vi "ADI_IMU_ADIS16448_ScaleData.vi"(4 "Received Data":u8[](array[numeric])) -> (1 "Data Array":dbl[](array[numeric]), 2 "Data Good?":bool)   [LabVIEW 2019, in "ADIS16448_IMU.lvlib"]
uses:
  ADIS16448_IMU.lvlib
panel:
  out "error out":errorcluster
  in  "error in (no error)":errorcluster
  out "Received CRC-16":u16
  out "Calculated CRC-16":u16
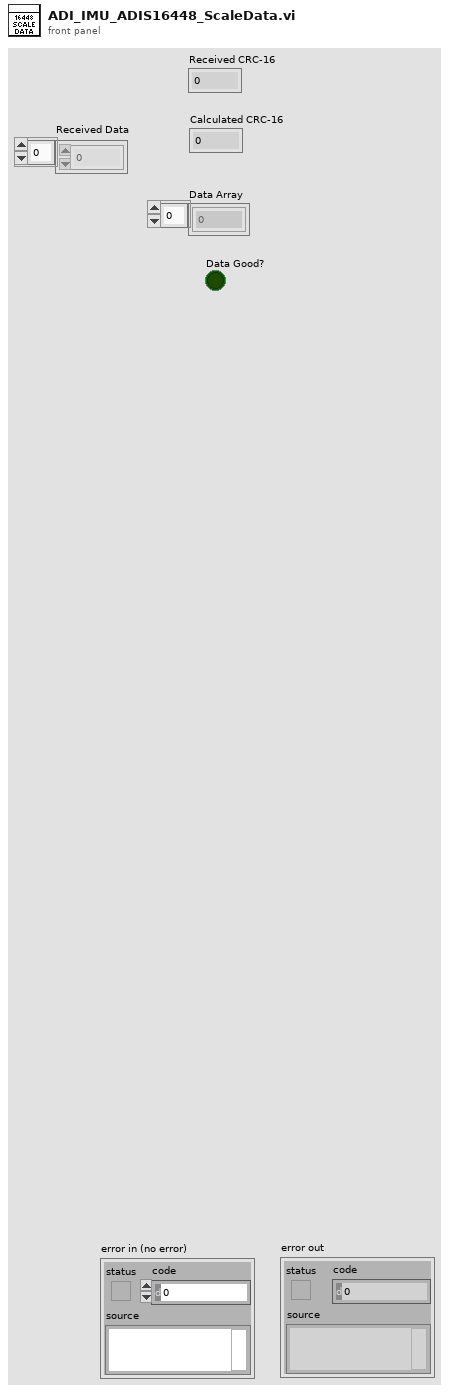
[diagram p1: front panel]
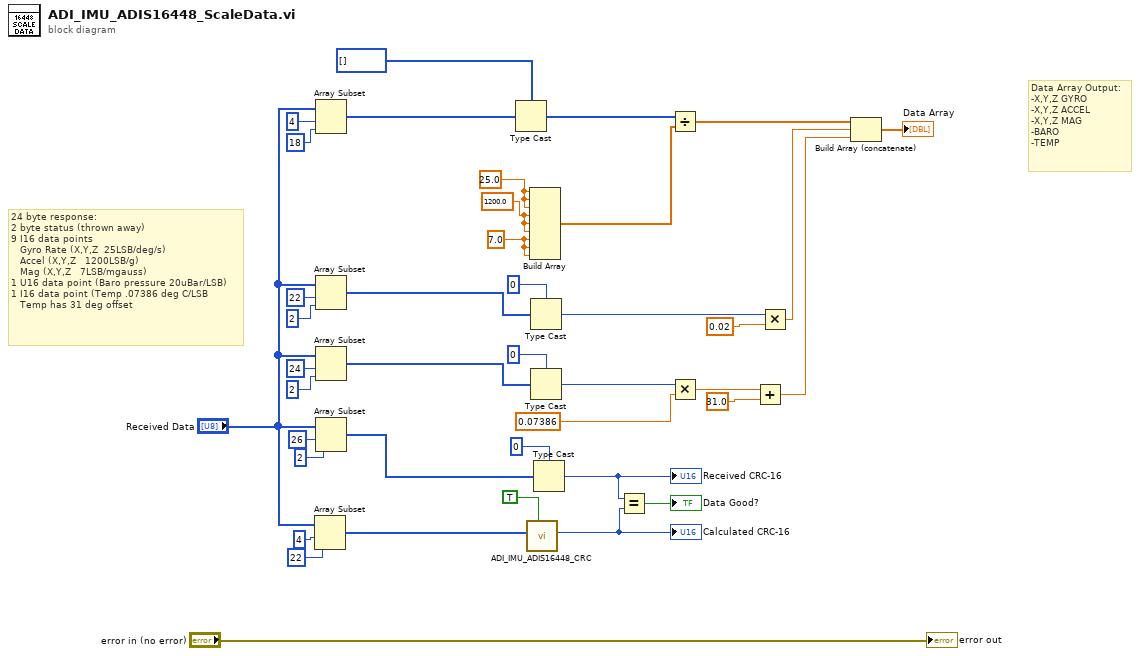
[diagram p0: block diagram]
diagram:
  w38 = 7.0
  w39 = 1200.0
  w40 = 25.0 ("element")
  # "Data Array Output:\n-X,Y,Z GYRO\n-X,Y,Z ACCEL\n-X,Y,Z MAG\n-BARO\n-TEMP"
  # "24 byte response:\n2 byte status (thrown away)\n9 I16 data points\n   Gyro Rate (X,Y,Z  25LSB/deg/s)\n   Accel (X,Y,Z   1200LSB/g)\n   Mag (X,Y,Z   7LSB/mgauss)\n1 U16 data point (Baro pressure 20uBar/LSB)\n1 I16 data point (Temp .07386 deg C/LSB\n   Temp has 31 deg offset"
  n1 = Array Subset(array="Received Data", index=4, length=22) -> (w5:u8[])
  n2 = Array Subset(array="Received Data", index=4, length=18) -> (w16:u8[])
  n3 = Array Subset(array="Received Data", index=22, length=2) -> (w22:u8[])
  n4 = Array Subset(array="Received Data", index=24, length=2) -> (w20:u8[])
  n5 = Array Subset(array="Received Data", index=26, length=2) -> (w10:u8[])
  n6 = Type Cast(type=i16[] [], x=w16) -> (*(type *) &x=w15:i16[])
  n7 = call "ADI_IMU_ADIS16448_CRC.vi"("Look-Up Table Method?"=TRUE, "Byte Array (MSB-First)"=w5) -> ("CRC16-ADIS"=w2:u16)  [unwired: 9 in]
  "Calculated CRC-16" <- w2
  n8 = Build Array(w40, w40, w40, w39, w39, w39, w38, w38, w38) -> (w37:dbl[])
  n9 = Type Cast(type=u16 0, x=w22) -> (*(type *) &x=w18:u16)
  n10 = Type Cast(type=i16 0, x=w20) -> (*(type *) &x=w17:i16)
  n11 = Type Cast(type=u16 0, x=w10) -> (*(type *) &x=w3:u16)
  "Received CRC-16" <- w3
  n12 = Equal?(x=w3, y=w2) -> (x = y?=→"Data Good?":bool)
  n13 = Divide(x=w15, y=w37) -> (x/y=w32:dbl[])
  n14 = Multiply(x=w17, y=0.07386 ("element")) -> (x*y=w34:dbl)
  n15 = Add(x=w34, y=31.0) -> (x+y=w31:dbl)
  n16 = Multiply(x=w18, y=0.02) -> (x*y=w29:dbl)
  n17 = Build Array (concatenate)(w32, w29, w31) -> (→"Data Array":dbl[])
  "error out" <- "error in (no error)"
